vi "withmic.vi"() -> ()   [LabVIEW 2019]
uses:
  <vilib>/sound2/lvsound2.llb/Sound File Refnum.ctl
  <vilib>/sound2/lvsound2.llb/Sound Data Format.ctl
  <vilib>/Analysis/baseanly.llb/Mean (DBL).vi
  <vilib>/Waveform/WDTOps.llb/WDT Waveform to XY Pairs DBL.vi
  <vilib>/express/express analysis/Spectral/Block/exnSpectralBlock spectral measurements RMS poly.vi
  <vilib>/express/express analysis/Spectral/Block/exnSpectralBlock spectral measurements RMS array WFM.vi
  <vilib>/express/express analysis/Spectral/Block/exnSpectralBlock spectral measurements RMS WFM.vi
  <vilib>/sound2/lvsound2.llb/Sound File Write Open.vi
  <vilib>/sound2/lvsound2.llb/Sound File Write (DBL Single).vi
  <vilib>/express/express analysis/Spectral/XNode/ExpressSpectralMeasurementsBlockNode.xnode
  <vilib>/Analysis/NI_AALBase.lvlib
  dllrt/Dll1/x64/Debug/Dll1.dll
panel:
  out "noisestd":dbl[](graph) caption="Data"
  out "noise type":string
  out "mean":dbl format="%0.2f"
  out "noisetype":dbl[](graph) caption="Data"
  out "energy":dbl[](graph) caption="Data"
  in  "Duration (s)":dbl=5.0
  in  "Sample rate (Hz)":dbl=44100.0
  in  "P":u64
  out "FFT Output":cluster{"f0":dbl, "df":dbl, "magnitude":dbl[]}(graph) caption="Data"
  out "FFT Input":cluster{"f0":dbl, "df":dbl, "magnitude":dbl[]}[](graph) caption="Data"
  in  "sound format":T1={"sample rate (S/s)"=22050.0, "number of channels"=2, "bits per sample"=16}
  in  "path 2":path
  out "sound file refnum":T2
  in  "Do you want to save?":bool
  in  "stop":bool
  in  "Device 2":u32 caption="Device"
  out "size(s)":i32
  out "Clean Output":waveform(dbl)(graph)
  out "Noisy Input":waveform(dbl)(graph)
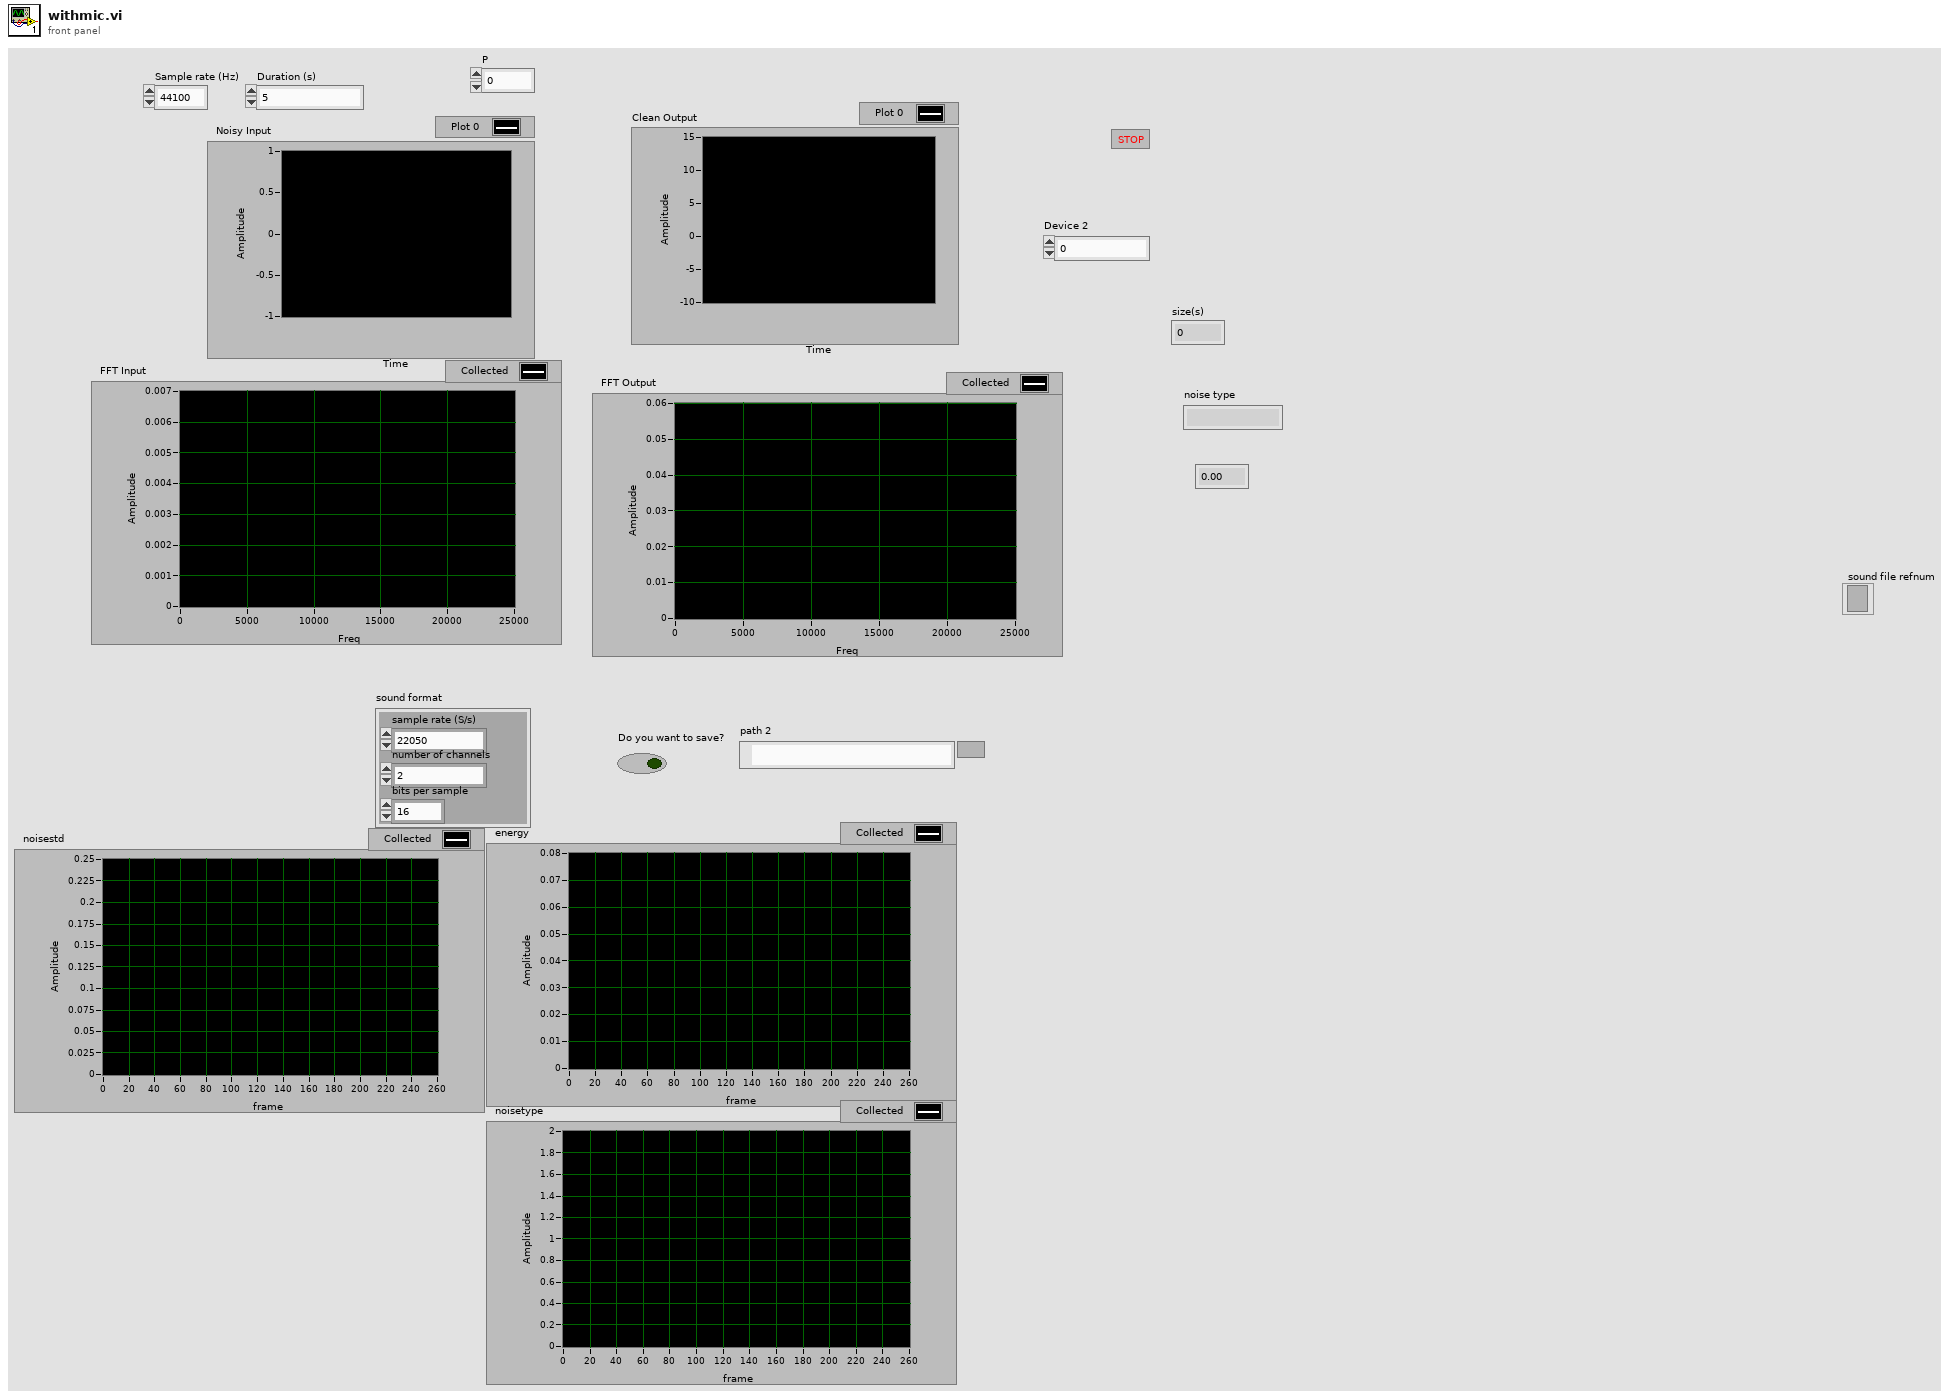
[diagram p1: front panel]
types:
  T1 = typedef "Sound Data Format.ctl" = cluster{"sample rate (S/s)":dbl, "number of channels":i32, "bits per sample":i32}
  T2 = typedef "Sound File Refnum.ctl" = refnum<file>
  T3 = cluster{"averaging mode":u16, "weighting mode":u16, "number of averages":u32}
  T4 = cluster{"dB On (F)":bool, "unwrap phase (F)":bool, "convert to degree (F)":bool}
  T5 = cluster{"Array of Waveform[0]":waveform(dbl), "Array of Waveform[1]":waveform(dbl), "Array of Waveform[2]":waveform(dbl), "Array of Waveform[3]":waveform(dbl), "Array of Waveform[4]":waveform(dbl), "Array of Waveform[5]":waveform(dbl), "Array of Waveform[6]":waveform(dbl), "Array of Waveform[7]":waveform(dbl), "Array of Waveform[8]":waveform(dbl)}
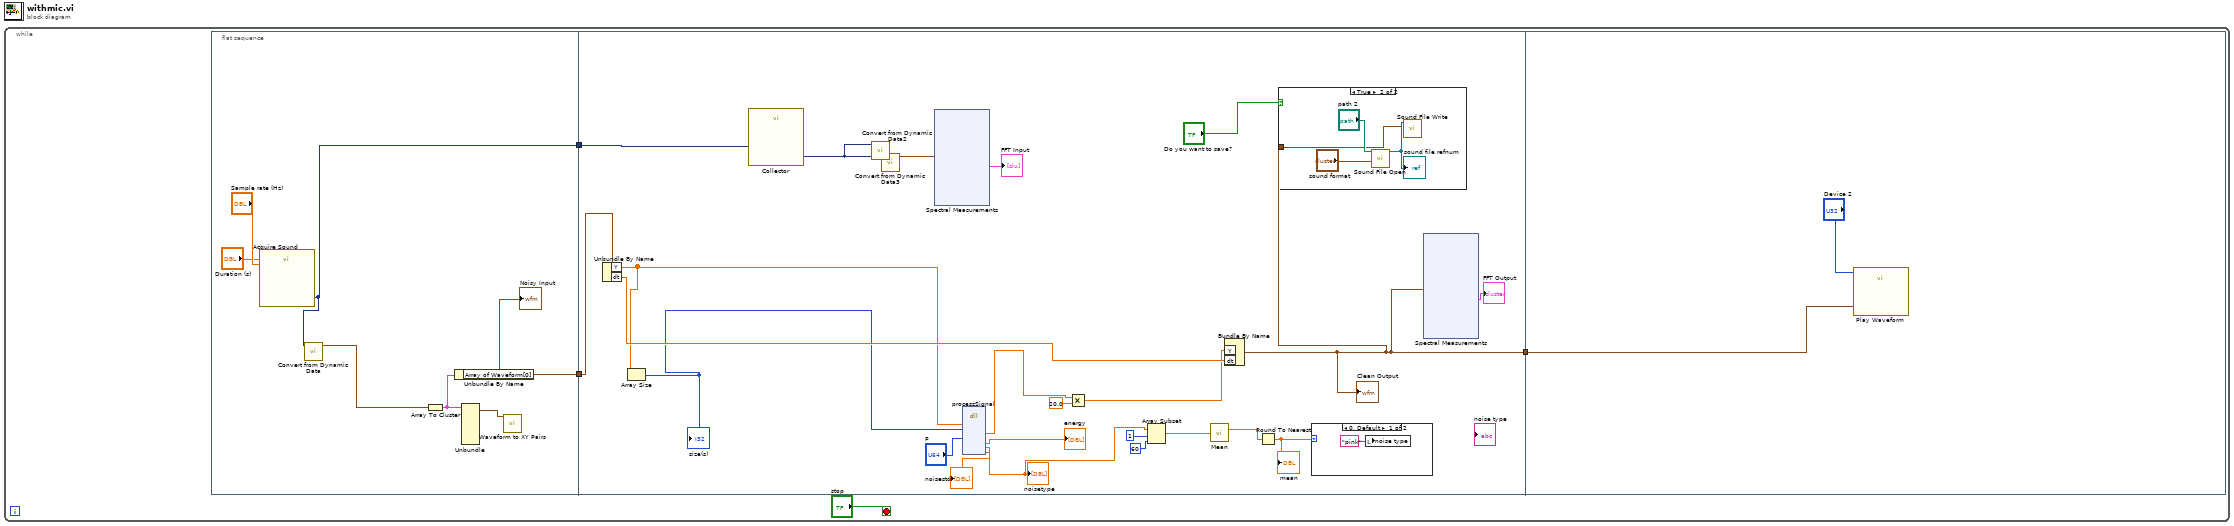
[diagram p0: block diagram]
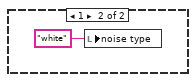
[diagram p2: hidden frame]
diagram:
  n1 = while {
    stop <- "stop" stop-if-true
    n2 = flat-sequence {
      tunnel: [w9] -> w3
      tunnel: [w7] -> w1
      tunnel: w3 -> [w34]
      tunnel: [w22] -> w2
      tunnel: w1 -> [w23]
      tunnel: w2 -> [w61]
      frame #0 {
        n3 = call "Acquire Sound"("Duration (s)"="Duration (s)", "Sample rate (Hz)"="Sample rate (Hz)") -> ("Data"=w7:dynamicdata)  [unwired: 16 in, 1 out]
        n4 = call "Convert from Dynamic Data"("Dynamic Data Type"=w7) -> ("Array of Waveform"=w8:waveform(dbl)[])  [unwired: 3 in]
        n5 = Array To Cluster(array=w8) -> (cluster=w10:T5)
        n6 = Unbundle By Name(w10) -> ("Array of Waveform[0]"=w9:waveform(dbl))
        "Noisy Input" <- w9
        n7 = Unbundle(w10) -> ("Array of Waveform[1]"=w11:waveform(dbl))  [unwired: 8 out]
        n8 = call-poly <vilib>:"Waveform to XY Pairs.vi"("waveform in"=w11) -> ()  [unwired: 8 in, 3 out]
      }
      frame #1 {
        n9 = Unbundle By Name(w34) -> ("Y"=w31:dbl[], "dt"=w33:dbl)
        n10 = Array Size(array=w31) -> (size(s)=w30:i32)
        "size(s)" <- w30
        n11 = call "Collector"("Signals"=w23) -> ("Collected Signals"=w26:dynamicdata)  [unwired: 9 in, 1 out]
        n12 = call "Convert from Dynamic Data2"("Dynamic Data Type"=w26) -> ()  [unwired: 3 in, 1 out]
        n13 = call "Convert from Dynamic Data3"("Dynamic Data Type"=w26) -> ("Array of Waveform"=w25:waveform(dbl)[])  [unwired: 3 in]
        n14 = xnode "Spectral Measurements"("Signals"=w25) -> ("FFT - (RMS)"=→"FFT Input":cluster{"f0":dbl, "df":dbl, "magnitude":dbl[]}[])  [unwired: 1 in, 2 out]
        n15 = dll-call lib="C:/Users/Yunus/Desktop/dllrt/Dll1/x64/Debug/Dll1.dll" fn="processSignal"("noisySignal"=w31, "signalLength"=w30, "P"="P") -> ("filteredSignal"=w29:dbl[], "speecher"=→"energy":dbl[], "noisetype"=w13:dbl[], "noisestd"=→"noisestd":dbl[])  [unwired: 11 in, 2 out]
        "noisetype" <- w13
        n16 = Multiply(x=w29, y=20.0) -> (x*y=w28:dbl[])
        n17 = Array Subset(array=w13, index=1, length=60) -> (w18:dbl[])
        n18 = call-poly <vilib>:"Mean.vi"("X"=w18) -> ("mean"=w16:dbl)  [unwired: 1 out]
        n19 = Bundle By Name("Y"=w28, "dt"=w33) -> (w22:waveform(dbl))  [unwired: 1 in]
        "Clean Output" <- w22
        n20 = Round To Nearest(number=w16) -> (nearest integer value=w17:dbl)
        "mean" <- w17
        n21 = case shown="True" "Do you want to save?" {
          tunnel: w22 -> [_ w57]
          frame False {
          }
          frame True {
            n22 = call-poly <vilib>:"Sound File Open.vi"("sound format"="sound format", "path"="path 2") -> ("sound file refnum"=w60:T2)  [unwired: 8 in, 1 out]
            "sound file refnum" <- w60
            n23 = call-poly <vilib>:"Sound File Write.vi"("data"=w57, "sound file refnum"=w60) -> ()  [unwired: 8 in, 2 out]
          }
        }
        n24 = case shown="0, Default" w17 {
          frame 0, Default {
            n25 = local write "noise type"("pink" ("String 2")) -> ()
          }
          frame 1 {
            n26 = local write "noise type"("white" ("String")) -> ()
          }
        }
        n27 = xnode "Spectral Measurements"("Signals"=w22) -> ("FFT - (RMS)"=→"FFT Output":cluster{"f0":dbl, "df":dbl, "magnitude":dbl[]})  [unwired: 1 in, 2 out]
      }
      frame #2 {
        n28 = call "Play Waveform"("Device"="Device 2", "Data"=w61) -> ()  [unwired: 17 in, 1 out]
      }
    }
  }
